vi "Set Defaults.vi"(11 "User in":refnum<class "User.lvclass">) -> (3 "User out":refnum<class "User.lvclass">)   [LabVIEW 2022 SP3, in "Conditum-Example.lvlib" / "User.lvclass"]
uses:
  User.lvclass
  User.lvclass/User.ctl
  Conditum/Columns/String/String.lvclass
  Conditum/Columns/Entity Collection/Entity Collection.lvclass
  Conditum/Columns/Integer/Integer.lvclass
  Conditum/Columns/Timestamp/Timestamp.lvclass
  Conditum/Columns/Boolean/Boolean.lvclass
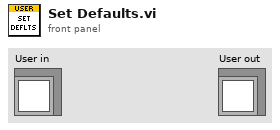
[diagram p1: front panel]
types:
  T1 = cluster{"Username":refnum<class "String.lvclass">, "Password":refnum<class "String.lvclass">, "Score":refnum<class "Integer.lvclass">, "Email":refnum<class "String.lvclass">, "Joined":refnum<class "Timestamp.lvclass">, "Has Logged In":refnum<class "Boolean.lvclass">, "Created Games":refnum<class "Entity Collection.lvclass">, "Joined Games":refnum<class "Entity Collection.lvclass">}
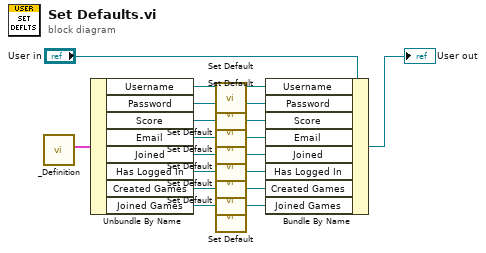
[diagram p0: block diagram]
diagram:
  n1 = call "_Definition.vi"() -> ("Definition"=w19:T1)  [unwired: 11 in]
  n2 = Unbundle By Name(w19) -> ("Username"=w18:refnum<class "String.lvclass">, "Password"=w16:refnum<class "String.lvclass">, "Score"=w15:refnum<class "Integer.lvclass">, "Email"=w14:refnum<class "String.lvclass">, "Joined"=w13:refnum<class "Timestamp.lvclass">, "Has Logged In"=w12:refnum<class "Boolean.lvclass">, "Created Games"=w11:refnum<class "Entity Collection.lvclass">, "Joined Games"=w17:refnum<class "Entity Collection.lvclass">)
  n3 = call-dynamic "Set Default.vi"("String in"=w18) -> ("String out"=w9:refnum<class "String.lvclass">)  [unwired: 10 in]
  n4 = call-dynamic "Set Default.vi"("String in"=w16) -> ("String out"=w8:refnum<class "String.lvclass">)  [unwired: 10 in]
  n5 = call-dynamic "Set Default.vi"("Integer in"=w15) -> ("Integer out"=w7:refnum<class "Integer.lvclass">)  [unwired: 10 in]
  n6 = call-dynamic "Set Default.vi"("String in"=w14) -> ("String out"=w6:refnum<class "String.lvclass">)  [unwired: 10 in]
  n7 = call-dynamic "Set Default.vi"("Timestamp in"=w13) -> ("Timestamp out"=w5:refnum<class "Timestamp.lvclass">)  [unwired: 10 in]
  n8 = call-dynamic "Set Default.vi"("Boolean in"=w12) -> ("Boolean out"=w4:refnum<class "Boolean.lvclass">)  [unwired: 10 in]
  n9 = call-dynamic "Set Default.vi"("Relation in"=w11) -> ("Relation out"=w3:refnum<class "Entity Collection.lvclass">)  [unwired: 10 in]
  n10 = call-dynamic "Set Default.vi"("Relation in"=w17) -> ("Relation out"=w2:refnum<class "Entity Collection.lvclass">)  [unwired: 10 in]
  n11 = Bundle By Name(cluster="User in", "Username"=w9, "Password"=w8, "Score"=w7, "Email"=w6, "Joined"=w5, "Has Logged In"=w4, "Created Games"=w3, "Joined Games"=w2) -> (→"User out":refnum<class "User.lvclass">)
